vi "FilterNaN.vi"(11 "input value":dbl) -> (3 "filtered value":dbl)   [LabVIEW 2017, in "McsaAnalysisFunctions.lvlib"]
uses:
  <vilib>/addons/InsightCM/Utilities/Analysis/MCSA/McsaAnalysisFunctions.lvlib
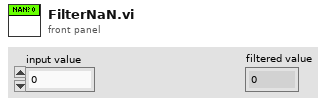
[diagram p1: front panel]
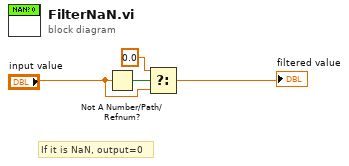
[diagram p0: block diagram]
diagram:
  # "If it is NaN, output=0"
  n1 = Not A Number/Path/Refnum?(number/path/refnum="input value") -> (NaN/Path/Refnum?=w1:bool)
  n2 = Select(t=0.0 ("x"), s=w1, f="input value") -> (s? t:f=→"filtered value":dbl)
